vi "PWRToggle.vi"(7 "PWRID":u8, 8 "error in (no error)":errorcluster {"code" format="%.0x"}, 9 "Channel":string="1", 10 "Enable Output (False)":bool, 11 "PWR In":refnum<visa-resource-name>) -> (0 "error out":errorcluster, 3 "PWR Out":refnum<visa-resource-name>)   [LabVIEW 2015]
uses:
  <instrlib>/Agilent N6700 Series/Agilent N6700 Series.lvlib
  <instrlib>/Agilent N87XX Series/Agilent N87XX Series.lvlib
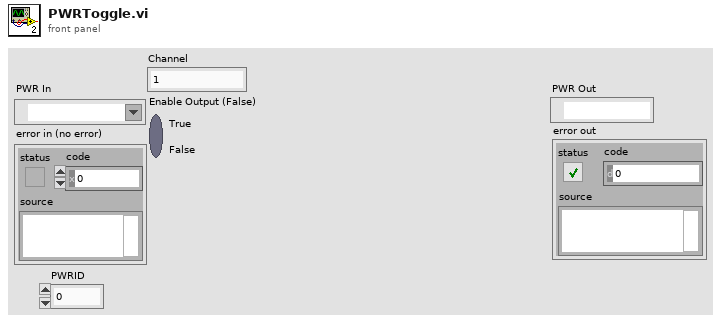
[diagram p1: front panel]
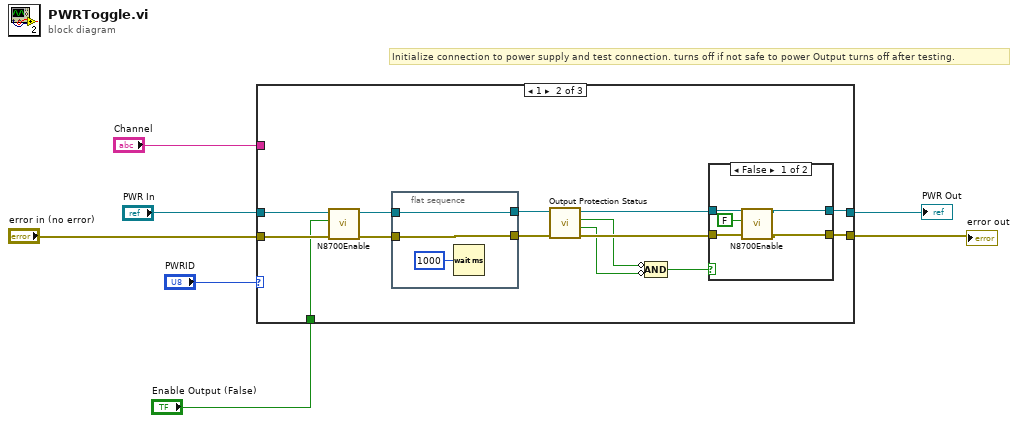
[diagram p0: block diagram]
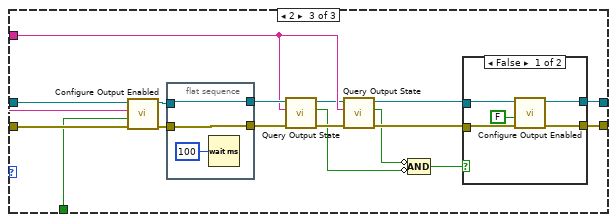
[diagram p4: hidden frame]
diagram:
  # "Initialize connection to power supply and test connection. turns off if not safe to power Output turns off after testing."
  n1 = case shown="1" "PWRID" {
    tunnel: [w9 w23 w48] -> w7
    tunnel: [w8 w22 w47] -> w6
    tunnel: "PWR In" -> [w9 w19 w46]
    tunnel: "error in (no error)" -> [w8 w18 w45]
    tunnel: "Channel" -> [_ _ w42]
    tunnel: "Enable Output (False)" -> [_ w17 w34]
    frame 0, Default {
    }
    frame 1 {
      n2 = call "N8700Enable.vi"("error in"=w18, "Enable Output (T: Enable)"=w17, "VISA resource name"=w19) -> ("error out"=w20:errorcluster, "VISA resource name out"=w21:refnum<visa-resource-name>)  [unwired: 7 in]
      n3 = flat-sequence {
        tunnel: w21 -> [w33]
        tunnel: [w33] -> w16
        tunnel: [w31] -> w15
        tunnel: w20 -> [w31]
        frame #0 {
          n4 = Wait (ms)(milliseconds to wait=u32 1000) -> ()  [unwired: 1 out]
        }
      }
      n5 = call <instrlib>:"Output Protection Status.vi"("error in (no error)"=w15, "VISA resource name"=w16) -> ("error out"=w13:errorcluster, "OCP Tripped?"=w11:bool, "OVP Tripped?"=w12:bool, "VISA resource name out"=w14:refnum<visa-resource-name>)  [unwired: 5 in, 1 out]
      n6 = Compound Arithmetic op=AND(invert w12, invert w11) -> (w10:bool)
      n7 = case shown="False" w10 {
        tunnel: w14 -> [w28 w30]
        tunnel: w13 -> [w27 w29]
        tunnel: [w26 w30] -> w23
        tunnel: [w25 w29] -> w22
        frame False {
          n8 = call "N8700Enable.vi"("error in"=w27, "Enable Output (T: Enable)"=FALSE, "VISA resource name"=w28) -> ("error out"=w25:errorcluster, "VISA resource name out"=w26:refnum<visa-resource-name>)  [unwired: 7 in]
        }
        frame True {
        }
      }
    }
    frame 2 {
      n9 = call <instrlib>:"Configure Output Enabled.vi"("error in (no error)"=w45, "Enable Output (False)"=w34, "Channel Name (1)"=w42, "VISA resource name"=w46) -> ("error out"=w49:errorcluster, "VISA resource name out"=w50:refnum<visa-resource-name>)  [unwired: 6 in]
      n10 = flat-sequence {
        tunnel: w50 -> [w60]
        tunnel: [w60] -> w44
        tunnel: [w58] -> w43
        tunnel: w49 -> [w58]
        frame #0 {
          n11 = Wait (ms)(milliseconds to wait=u32 100) -> ()  [unwired: 1 out]
        }
      }
      n12 = call <instrlib>:"Query Output State.vi"("error in (no error)"=w43, "Channel Name (1)"=w42, "VISA resource name"=w44) -> ("error out"=w40:errorcluster, "In State"=w36:bool, "VISA resource name out"=w41:refnum<visa-resource-name>)  [unwired: 6 in]
      n13 = call <instrlib>:"Query Output State.vi"("error in (no error)"=w40, "Channel Name (1)"=w42, "VISA resource name"=w41) -> ("error out"=w39:errorcluster, "In State"=w37:bool, "VISA resource name out"=w38:refnum<visa-resource-name>)  [unwired: 6 in]
      n14 = Compound Arithmetic op=AND(invert w37, invert w36) -> (w35:bool)
      n15 = case shown="False" w35 {
        tunnel: w38 -> [w55 w57]
        tunnel: w39 -> [w54 w56]
        tunnel: [w52 w57] -> w48
        tunnel: [w51 w56] -> w47
        frame False {
          n16 = call <instrlib>:"Configure Output Enabled.vi"("error in (no error)"=w54, "Enable Output (False)"=FALSE, "VISA resource name"=w55) -> ("error out"=w51:errorcluster, "VISA resource name out"=w52:refnum<visa-resource-name>)  [unwired: 7 in]
        }
        frame True {
        }
      }
    }
  }
  "PWR Out" <- w7
  "error out" <- w6
